vi "ReadChannelFromNanoVoltMeter.vi"(11 "ChannelSelection":dbl) -> (1 "String Measurement":string, 2 "error out":errorcluster, 3 "Measurement":dbl)   [LabVIEW 2009]
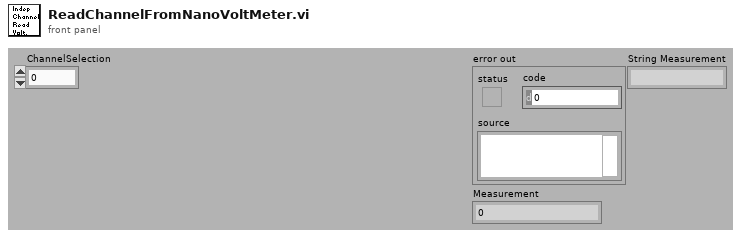
[diagram p1: front panel]
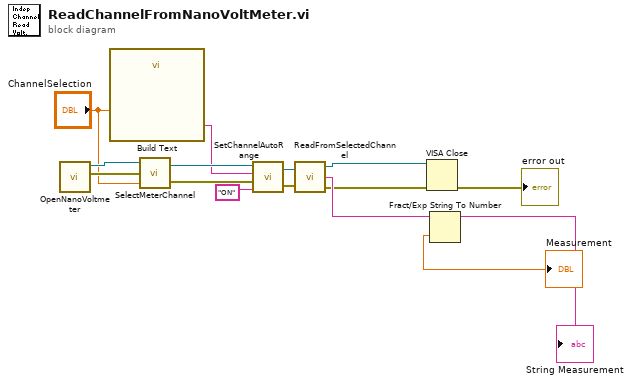
[diagram p0: block diagram]
diagram:
  n1 = call "OpenNanoVoltmeter.vi"() -> ("error out"=w13:errorcluster, "reference out"=w14:refnum<visa-resource-name>)  [unwired: 8 in]
  n2 = call "Build Text"("channel"="ChannelSelection") -> ("Result"=w8:string)  [unwired: 13 in, 1 out]
  n3 = call "SelectMeterChannel.vi"("ChannelSelection"="ChannelSelection", "error out"=w13, "reference out"=w14) -> ("error out 2"=w11:errorcluster, "reference out 2"=w12:refnum<visa-resource-name>)
  n4 = call "SetChannelAutoRange.vi"("On/Off"="ON", "error out 2"=w11, "Channel"=w8, "reference out 2"=w12) -> ("error out"=w6:errorcluster, "reference out 3"=w7:refnum<visa-resource-name>)
  n5 = call "ReadFromSelectedChannel.vi"("reference out 3"=w7, "error out"=w6) -> ("reference out 4"=w4:refnum<visa-resource-name>, "read buffer"=w5:string, "error out 2"=w3:errorcluster)
  "String Measurement" <- w5
  n6 = VISA Close(VISA resource name=w4, error in (no error)=w3) -> (error out=→"error out":errorcluster)
  n7 = Fract/Exp String To Number(string=w5) -> (number=→"Measurement":dbl)  [unwired: 3 in, 1 out]
